vi "test.vi"() -> ()   [LabVIEW 2019]
uses:
  Source/Shared/DeltaPSControl Shared.lvlib
  Source/Engine/DeltaPSControl Engine.lvlib
panel:
  out "Reg B":i16[](array[numeric])
  out "Reg A":i16[](array[numeric])
  out "number 4":dbl
  out "number 3":dbl
  out "number 2":dbl
  out "number":dbl
  out "error out":errorcluster
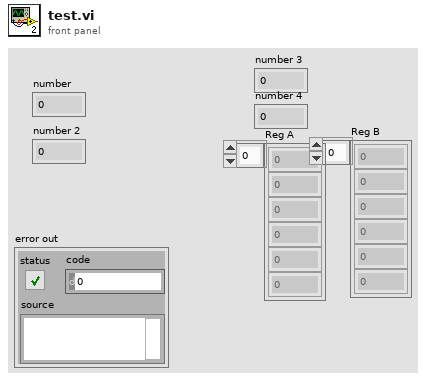
[diagram p1: front panel]
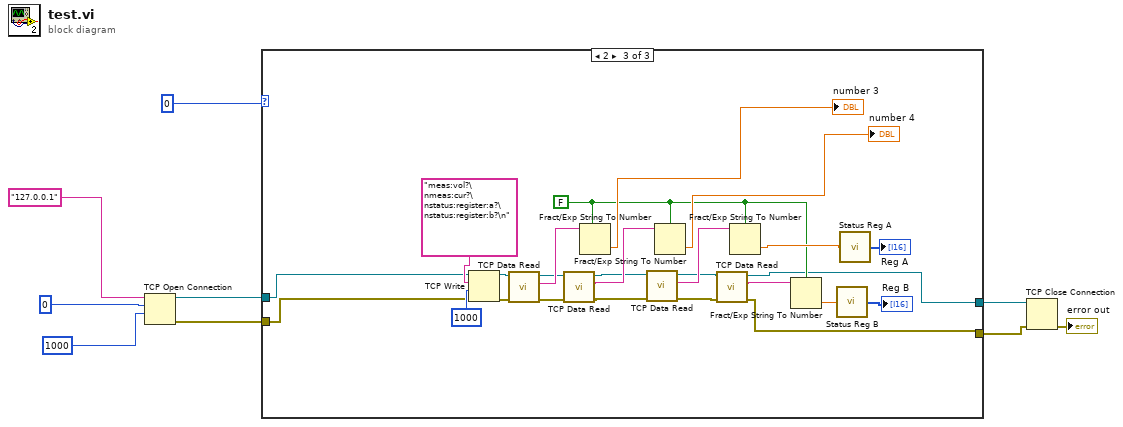
[diagram p0: block diagram]
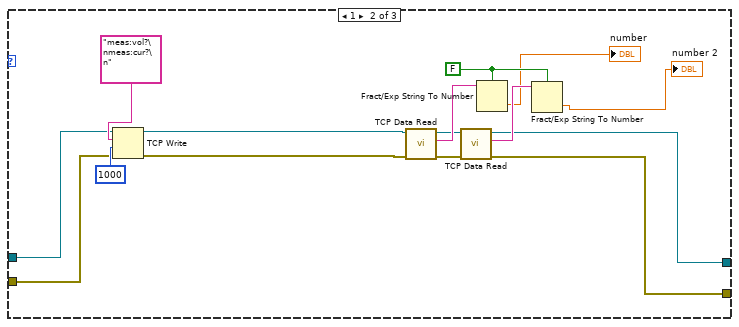
[diagram p3: hidden frame]
diagram:
  n1 = TCP Open Connection(address="127.0.0.1", remote port or service name=u16 0 ("Port"), timeout ms (60000)=1000) -> (connection ID=w5:refnum<k5>, error out=w2:errorcluster)  [unwired: 2 in]
  n2 = case shown="2" 0 {
    tunnel: w5 -> [w11 w19 w32]
    tunnel: [w11 w13 w30] -> w4
    tunnel: [w10 w12 w29] -> w3
    tunnel: w2 -> [w10 w18 w31]
    frame 0, Default {
    }
    frame 1 {
      w17 = FALSE ("use system decimal point (T)")
      n3 = TCP Write(connection ID=w19, data in="meas:vol?\nmeas:cur?\n", error in (no error)=w18, 9:1000) -> (connection ID out=w26:refnum<k5>, error out=w25:errorcluster)  [unwired: 1 out]
      n4 = call "TCP Data Read.vi"("error in (no error)"=w25, "Connection ID in"=w26) -> ("error out"=w22:errorcluster, "TCP Read data"=w24:string, "Connection ID out"=w23:refnum<k5>)  [unwired: 6 in, 1 out]
      n5 = call "TCP Data Read.vi"("error in (no error)"=w22, "Connection ID in"=w23) -> ("error out"=w12:errorcluster, "TCP Read data"=w16:string, "Connection ID out"=w13:refnum<k5>)  [unwired: 6 in, 1 out]
      n6 = Fract/Exp String To Number(use system decimal point (T)=w17, string=w24) -> (number=→"number":dbl)  [unwired: 2 in, 1 out]
      n7 = Fract/Exp String To Number(use system decimal point (T)=w17, string=w16) -> (number=→"number 2":dbl)  [unwired: 2 in, 1 out]
    }
    frame 2 {
      w33 = FALSE ("use system decimal point (T)")
      n8 = TCP Write(connection ID=w32, data in="meas:vol?\nmeas:cur?\nstatus:register:a?\nstatus:register:b?\n", error in (no error)=w31, 9:1000) -> (connection ID out=w49:refnum<k5>, error out=w48:errorcluster)  [unwired: 1 out]
      n9 = call "TCP Data Read.vi"("error in (no error)"=w48, "Connection ID in"=w49) -> ("error out"=w45:errorcluster, "TCP Read data"=w47:string, "Connection ID out"=w46:refnum<k5>)  [unwired: 6 in, 1 out]
      n10 = call "TCP Data Read.vi"("error in (no error)"=w45, "Connection ID in"=w46) -> ("error out"=w42:errorcluster, "TCP Read data"=w44:string, "Connection ID out"=w43:refnum<k5>)  [unwired: 6 in, 1 out]
      n11 = Fract/Exp String To Number(use system decimal point (T)=w33, string=w47) -> (number=→"number 3":dbl)  [unwired: 2 in, 1 out]
      n12 = call "TCP Data Read.vi"("error in (no error)"=w42, "Connection ID in"=w43) -> ("error out"=w39:errorcluster, "TCP Read data"=w41:string, "Connection ID out"=w40:refnum<k5>)  [unwired: 6 in, 1 out]
      n13 = Fract/Exp String To Number(use system decimal point (T)=w33, string=w44) -> (number=→"number 4":dbl)  [unwired: 2 in, 1 out]
      n14 = call "TCP Data Read.vi"("error in (no error)"=w39, "Connection ID in"=w40) -> ("error out"=w29:errorcluster, "TCP Read data"=w38:string, "Connection ID out"=w30:refnum<k5>)  [unwired: 6 in, 1 out]
      n15 = Fract/Exp String To Number(use system decimal point (T)=w33, string=w41) -> (number=w37:dbl)  [unwired: 2 in, 1 out]
      n16 = Fract/Exp String To Number(use system decimal point (T)=w33, string=w38) -> (number=w36:dbl)  [unwired: 2 in, 1 out]
      n17 = call "Status Reg B.vi"("Status:Register:B"=w36) -> ("Reg B"=→"Reg B":i16[])
      n18 = call "Status Reg A.vi"("Status:Register:A"=w37) -> ("Reg A"=→"Reg A":i16[])
    }
  }
  n19 = TCP Close Connection(connection ID=w4, error in (no error)=w3) -> (error out=→"error out":errorcluster)  [unwired: 1 in, 1 out]
